vi "launch IE.vi"(8 "error in (no error)":errorcluster, 11 "web site":string) -> (0 "error out":errorcluster)   [LabVIEW 2019]
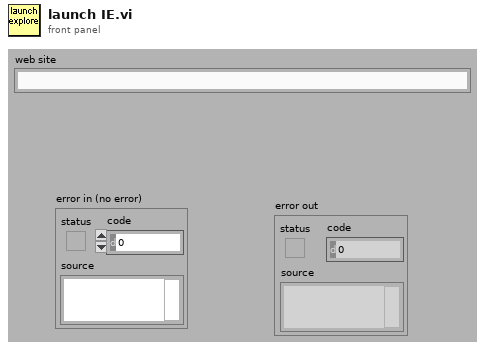
[diagram p1: front panel]
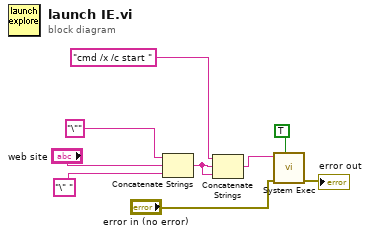
[diagram p0: block diagram]
diagram:
  n1 = Concatenate Strings("\"" ("Substring"), "web site", "\" " ("Substring")) -> (w5:string)
  n2 = Concatenate Strings("cmd /x /c start ", w5, w5) -> (w3:string)
  n3 = call <vilib>:"System Exec.vi"("wait until completion? (T)"=TRUE ("Wait until done"), "error in (no error)"="error in (no error)", "command line"=w3) -> ("error out"=→"error out":errorcluster)  [unwired: 5 in, 3 out]
